vi "GOOP_LVClass_Provider_NotifyChanged.vi"(10 "Change Type":T1=enum."Item Modified", 11 "Object":u64[](array[numeric]) caption="item IDs") -> ()   [LabVIEW 2012]
uses:
  <resource>/Framework/Providers/API/mxLvChangeType.ctl
  <resource>/Framework/Providers/Open_GDS/ClassProviders/Provider_BaseClassInterface/ClassWriter_class/ClassWriter.lvclass
  <resource>/Framework/Providers/Open_GDS/SubVIs/GOOP_ClassProviderClassType.ctl
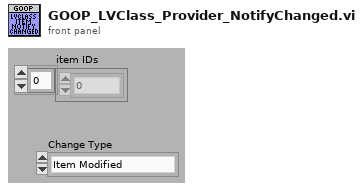
[diagram p1: front panel]
types:
  T1 = typedef "mxLvChangeType.ctl" = enum32{"Item Created", "Item Modified", "File Modified", "File Deleted", "Item Added", "Item Added to SCC", "Item Renamed", "Item Modified For SCC"}
  T2 = typedef "GOOP_ClassProviderClassType.ctl" = enum16{"ClassWriter", "ClassReader"}
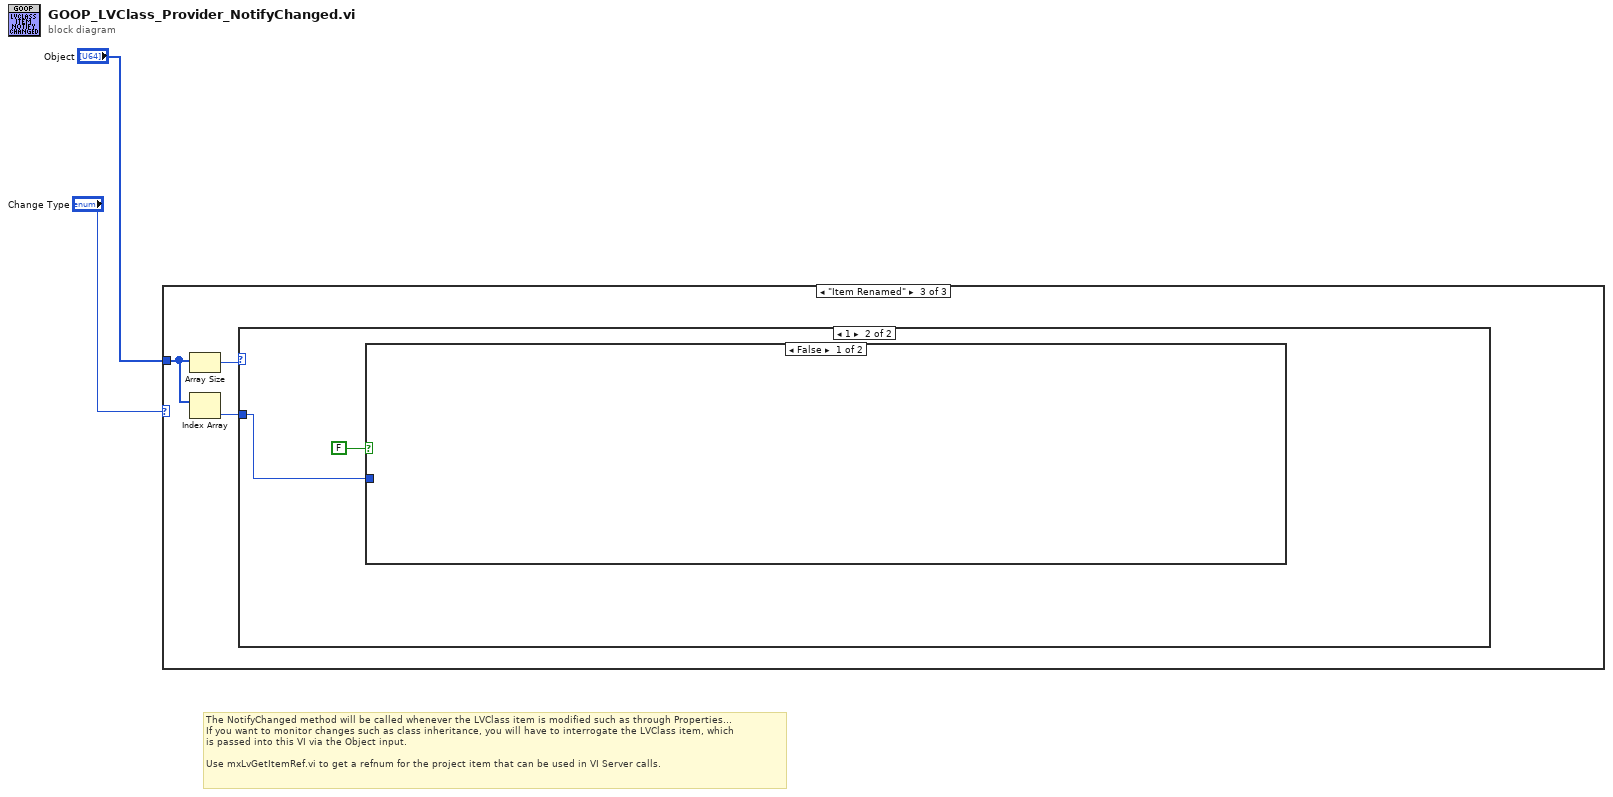
[diagram p0: block diagram]
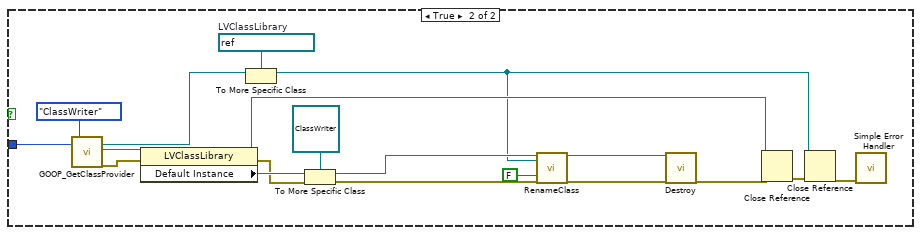
[diagram p5: hidden frame]
diagram:
  # "The NotifyChanged method will be called whenever the LVClass item is modified such as through Properties...\nIf you want to monitor changes such as class inheritance, you will have to interrogate the LVClass item, which\nis passed into this VI via the Object input.\n\nUse mxLvGetItemRef.vi to get a refnum for the project item that can be used in VI Server calls."
  n1 = case shown="\"Item Renamed\"" "Change Type" {
    tunnel: "Object" -> [_ _ w4]
    frame "Item Created", Default {
    }
    frame "Item Modified" {
    }
    frame "Item Renamed" {
      n2 = Array Size(array=w4) -> (size(s)=w5:i32)
      n3 = Index Array(array=w4) -> (element=w3:u64)  [unwired: 1 in]
      n4 = case shown="1" w5 {
        tunnel: w3 -> [_ w7]
        frame 0, Default {
        }
        frame 1 {
          n5 = case shown="False" FALSE {
            tunnel: w7 -> [_ w26]
            frame False {
            }
            frame True {
              w16 = refnum<vi> refnum  # LVClassLibrary
              n6 = call <resource>:"GOOP_GetClassProvider.vi"("New Item Parent/Object"=w26, "ProviderClassType"=GOOP_ClassProviderClassType."ClassWriter") -> ("ProjectItem"=w17:refnum<vi>, "LVClass.Open"=w15:refnum<vi>, "error out"=w21:errorcluster)  [unwired: 15 in]
              n7 = property class="LVClassLibrary"(reference=w15, error in=w21) -> (reference out=w19:refnum<vi>, error out=w24:errorcluster, "Default Instance"=w25:refnum<class>)
              n8 = To More Specific Class(target class=w16, reference=w17) -> (specific class reference=w9:refnum<vi>)  [unwired: 1 in, 1 out]
              n9 = To More Specific Class(target class=refnum<class "ClassWriter.lvclass"> refnum ("ClassWriter.lvclass"), reference=w25, error in=w24) -> (specific class reference=w13:refnum<class "ClassWriter.lvclass">, error out=w10:errorcluster)
              n10 = call-dynamic "RenameClass.vi"("ClassWriter.lvclass"=w13, "ClassRef"=w9, "RelinkWholeProject"=FALSE, "error in (no error)"=w10) -> ("ClassWriter.lvclass"=w12:refnum<class "ClassWriter.lvclass">, "error out"=w11:errorcluster)  [unwired: 14 in]
              n11 = call-dynamic "Destroy.vi"("ClassWriter.lvclass"=w12, "error in (no error)"=w11) -> ("error out"=w14:errorcluster)  [unwired: 17 in]
              n12 = Close Reference(reference=w19, error in (no error)=w14) -> (error out=w23:errorcluster)
              n13 = Close Reference(reference=w9, error in (no error)=w23) -> (error out=w22:errorcluster)
              n14 = call <vilib>:"Simple Error Handler.vi"("error in (no error)"=w22) -> ()  [unwired: 4 in, 5 out]
            }
          }
        }
      }
    }
  }
